vi "TemperaturRegler.vi"(6 "error in":errorcluster, 8 "TemperaturReglerEigenschaftenIn":T1, 9 "ZielTemperatur":dbl, 10 "AktTemperatur":dbl, 11 "AktiverReglerNr":u8) -> (0 "TemperaturReglerEigenschaftenOut":T1, 3 "Ventilstellung":dbl, 4 "error out":errorcluster)   [LabVIEW 2024]
doc: "Dieses VI steuert die Temperatur je anch Eingangsbelegung auf Basis einen PID- oder 2 Punkt Reglers.\nEs muss zyklisch aufgerufen werden.\nIst der 2 Punkt Rgeler aktiv werden die PID-Eigenschaften 1:1 wieder ausgegeben.\nPID-Eigenschaften Out un In unterscheiden sich iniherer Bedeutung.\nz.B.: PID-Eigenschaften-In.AutoTune gibt an das der PID Regler sich selbst justeiren soll. PID-Eigenschaften-Out.AutoTune gibt an ob er mit der Selbstjustierung fertig ist."
uses:
  TemperaturReglerEigenschaften.ctl
  3PunktreglerEigenschaften.ctl
  PIDEigenschaften.ctl
  PIDRegelparameter.ctl
  <vilib>/addons/control/pid/NI_PID_autopid.lvlib
panel:
  # "Bei 0 ist PID-Rgeler Aktiv, bei 1 der 2 Punkt-Regler"
  # "in Grad"
  # "in %"
  # "in %"
  # "in Grad"
  # "in %"
  # "in %"
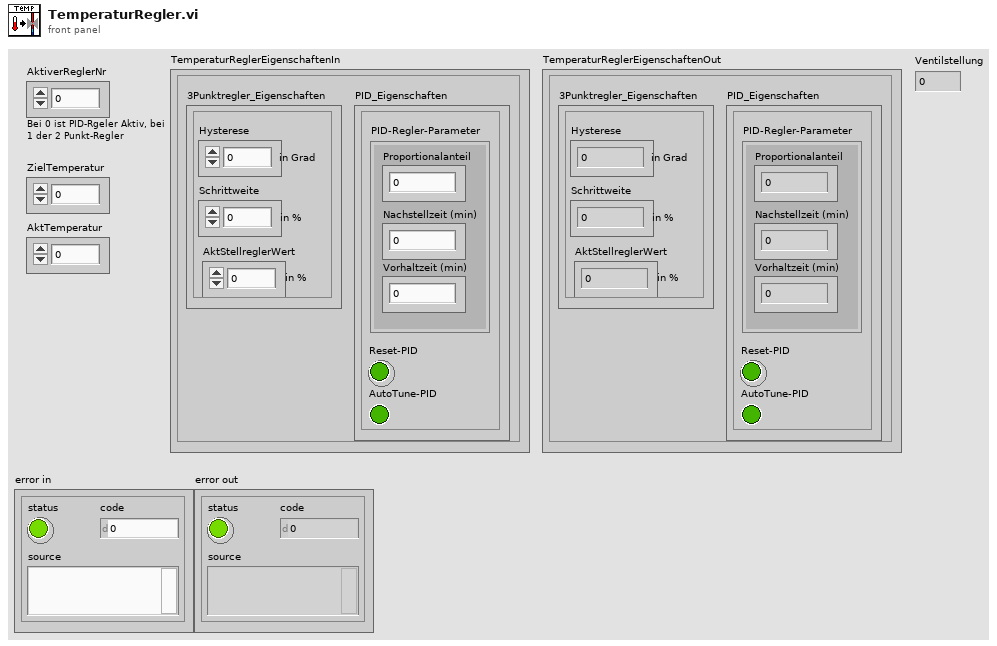
[diagram p1: front panel]
types:
  T1 = typedef "TemperaturReglerEigenschaften.ctl" = cluster{"3Punktregler_Eigenschaften":T2, "PID_Eigenschaften":T3}
  T2 = typedef "3PunktreglerEigenschaften.ctl" = cluster{"Hysterese":dbl, "Schrittweite":dbl, "AktStellreglerWert":dbl}
  T3 = typedef "PIDEigenschaften.ctl" = cluster{"PID-Regler-Parameter":T4, "Reset-PID":bool, "AutoTune-PID":bool}
  T4 = typedef "PIDRegelparameter.ctl" = cluster{"Nachstellzeit (min)":dbl, "Vorhaltzeit (min)":dbl, "Proportionalanteil":dbl}
  T5 = cluster{"process gain":dbl, "time constant (s)":dbl, "delay time (s)":dbl}
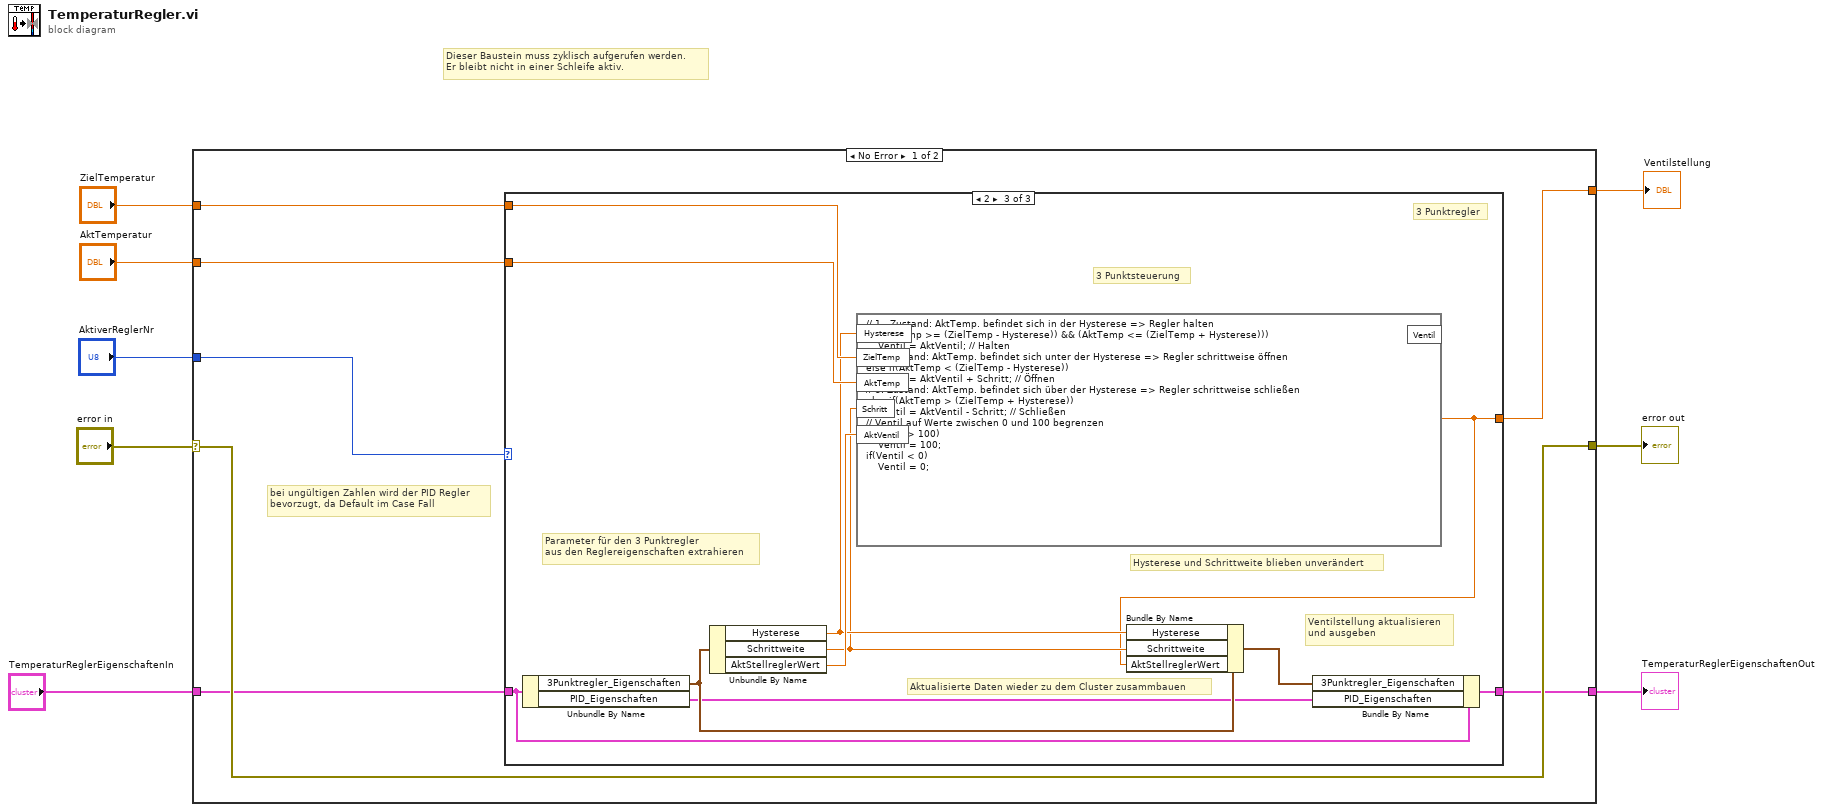
[diagram p0: block diagram]
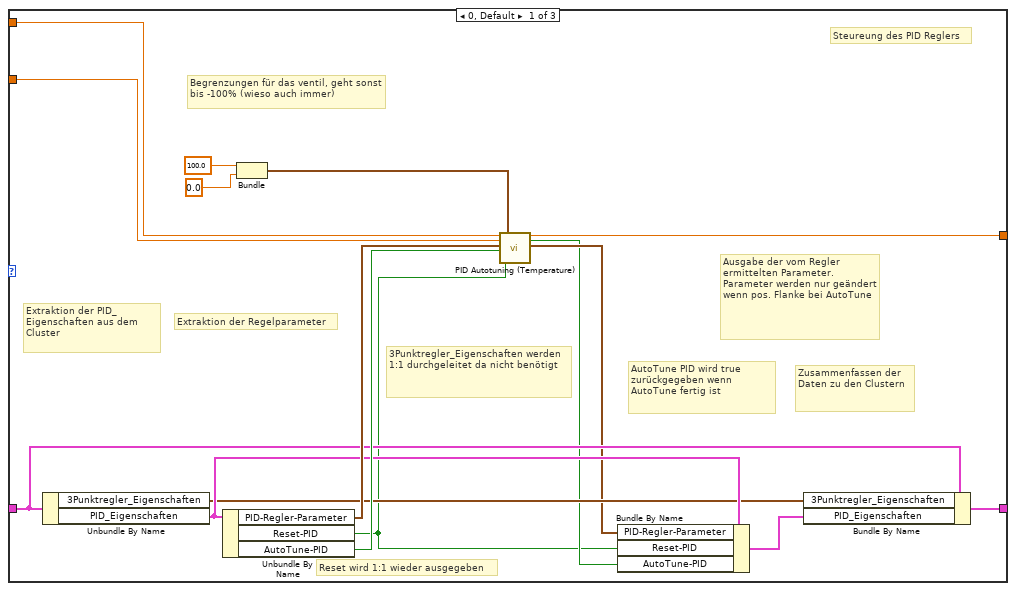
[diagram p2: hidden frame]
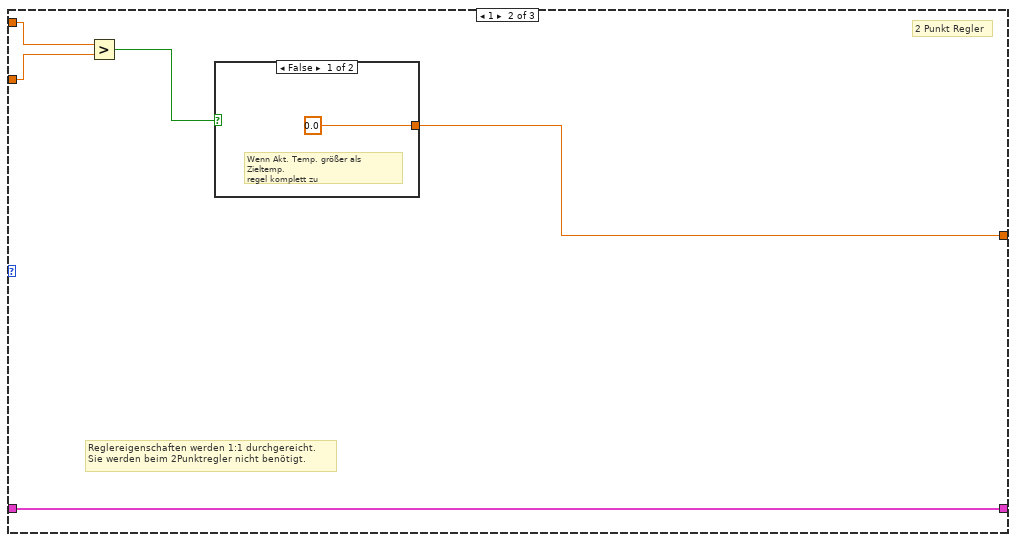
[diagram p3: hidden frame]
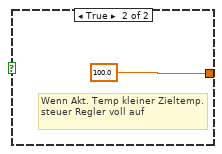
[diagram p4: hidden frame]
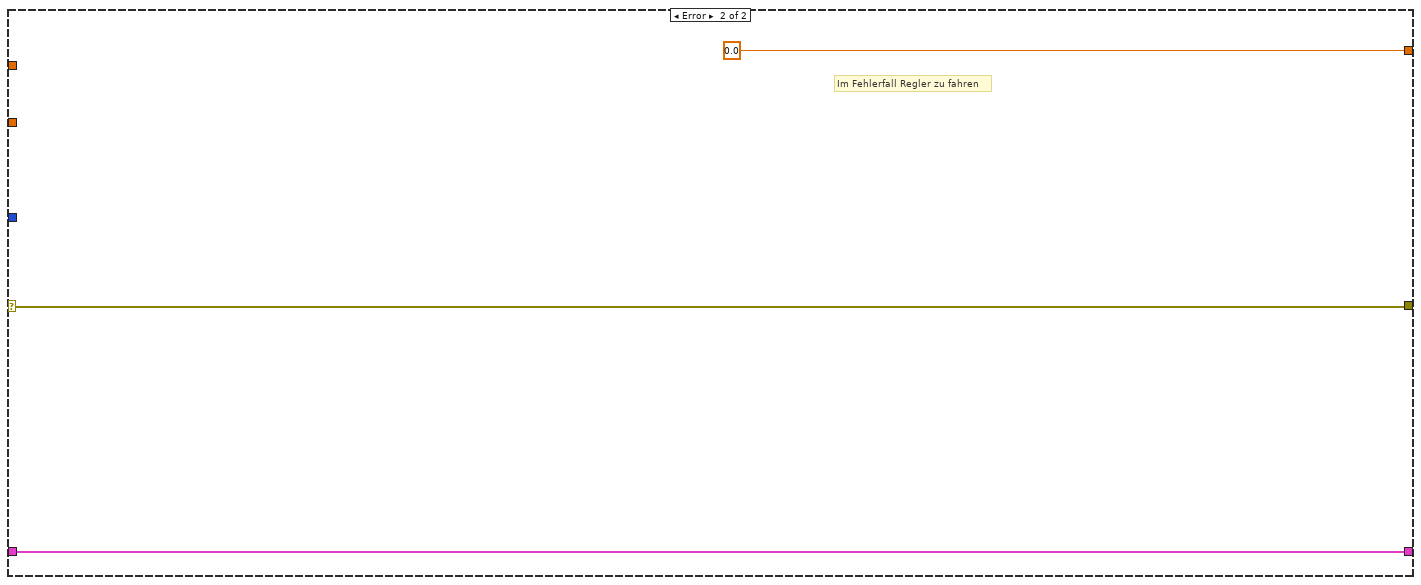
[diagram p5: hidden frame]
diagram:
  # "Dieser Baustein muss zyklisch aufgerufen werden.\nEr bleibt nicht in einer Schleife aktiv."
  n1 = case shown="No Error" "error in" {
    selector: "error in" -> [w15 w52]
    tunnel: [w15 w52] -> w7
    tunnel: "ZielTemperatur" -> [w14 _]
    tunnel: [w11 0.0] -> w5
    tunnel: "TemperaturReglerEigenschaftenIn" -> [w13 w50]
    tunnel: "AktTemperatur" -> [w12 _]
    tunnel: [w10 w50] -> w1
    tunnel: "AktiverReglerNr" -> [w9 _]
    frame No Error {
      # "bei ungültigen Zahlen wird der PID Regler\nbevorzugt, da Default im Case Fall"
      n2 = case shown="2" w9 {
        tunnel: w14 -> [w28 w35 w49]
        tunnel: w13 -> [w23 w36 w46]
        tunnel: w12 -> [w27 w34 w47]
        tunnel: [w26 w32 w40] -> w11
        tunnel: [w19 w36 w45] -> w10
        frame 0, Default {
          # "Zusammenfassen der Daten zu den Clustern"
          # "AutoTune PID wird true zurückgegeben wenn AutoTune fertig ist"
          # "Ausgabe der vom Regler ermittelten Parameter.\nParameter werden nur geändert wenn pos. Flanke bei AutoTune"
          # "Extraktion der Regelparameter"
          # "Extraktion der PID_Eigenschaften aus dem Cluster"
          # "3Punktregler_Eigenschaften werden 1:1 durchgeleitet da nicht benötigt"
          # "Reset wird 1:1 wieder ausgegeben"
          # "Begrenzungen für das ventil, geht sonst bis -100% (wieso auch immer)"
          # "Steureung des PID Reglers"
          n3 = Unbundle By Name(w23) -> ("3Punktregler_Eigenschaften"=w20:T2, "PID_Eigenschaften"=w22:T3)
          n4 = Unbundle By Name(w22) -> ("PID-Regler-Parameter"=w25:T4, "Reset-PID"=w16:bool, "AutoTune-PID"=w24:bool)
          n5 = Bundle(100.0, 0.0) -> (w29:cluster{dbl, dbl})  [unwired: 1 in]
          n6 = call <vilib>:"PID Autotuning (Temperature).vi"("desired temperature"=w28, "measured temperature"=w27, "plant parameters in"=w25, "autotune? (F)"=w24, "output range"=w29, "reinitialize? (F)"=w16) -> ("output"=w26:dbl, "tuning completed?"=w17:bool, "plant parameters out"=w18:T5)  [unwired: 10 in, 1 out]
          n7 = Bundle By Name(cluster=w22, "PID-Regler-Parameter"=w18, "Reset-PID"=w16, "AutoTune-PID"=w17) -> (w21:T3)
          n8 = Bundle By Name(cluster=w23, "3Punktregler_Eigenschaften"=w20, "PID_Eigenschaften"=w21) -> (w19:T1)
        }
        frame 1 {
          # "Reglereigenschaften werden 1:1 durchgereicht.\nSie werden beim 2Punktregler nicht benötigt."
          # "2 Punkt Regler"
          n9 = Greater?(x=w35, y=w34) -> (0:w33:bool)
          n10 = case shown="False" w33 {
            tunnel: [0.0 100.0] -> w32
            frame False {
              # "Wenn Akt. Temp. größer als Zieltemp.\nregel komplett zu"
            }
            frame True {
              # "Wenn Akt. Temp kleiner Zieltemp. steuer Regler voll auf"
            }
          }
        }
        frame 2 {
          # "3 Punktsteuerung"
          # "Aktualisierte Daten wieder zu dem Cluster zusammbauen"
          # "Ventilstellung aktualisieren \nund ausgeben"
          # "Hysterese und Schrittweite blieben unverändert"
          # "Parameter für den 3 Punktregler\naus den Reglereigenschaften extrahieren"
          # "3 Punktregler"
          n11 = Unbundle By Name(w46) -> ("3Punktregler_Eigenschaften"=w44:T2, "PID_Eigenschaften"=w39:T3)
          n12 = Unbundle By Name(w44) -> ("Hysterese"=w42:dbl, "Schrittweite"=w41:dbl, "AktStellreglerWert"=w48:dbl)
          n13 = formula code="// 1.  Zustand: AktTemp. befindet sich in der Hysterese => Regler halten\nif((AktTemp >= (ZielTemp - Hysterese)) && (AktTemp <= (ZielTemp + Hysterese))) \n    Ventil = AktVentil; // Halten\n// 2. Zustand: AktTemp. befindet sich unter der Hysterese => Regler schrittweise öffnen\nelse if(AktTemp < (ZielTemp - Hysterese)) \n    Ventil = AktVentil + Schritt; // Öffnen\n// 3. Zustand: AktTemp. befindet sich über der Hysterese => Regler schrittweise schließen\nelse if(AktTemp > (ZielTemp + Hysterese)) \n    Ventil = AktVentil - Schritt; // Schließen\n// Ventil auf Werte zwischen 0 und 100 begrenzen\nif(Ventil > 100)\n    Ventil = 100;\nif(Ventil < 0)\n    Ventil = 0;"("Hysterese"=w42, "ZielTemp"=w49, "AktTemp"=w47, "Schritt"=w41, "AktVentil"=w48) -> ("Ventil"=w40:dbl)
          n14 = Bundle By Name(cluster=w44, "Hysterese"=w42, "Schrittweite"=w41, "AktStellreglerWert"=w40) -> (w43:T2)
          n15 = Bundle By Name(cluster=w46, "3Punktregler_Eigenschaften"=w43, "PID_Eigenschaften"=w39) -> (w45:T1)
        }
      }
    }
    frame Error {
      # "Im Fehlerfall Regler zu fahren"
    }
  }
  "error out" <- w7
  "Ventilstellung" <- w5
  "TemperaturReglerEigenschaftenOut" <- w1
